vi "Teleop.vi"(10 "Match Info":T4={"Autonomous Elapsed Seconds"=0.0, "TeleOp Elapsed Seconds"=0.0, "Disabled Elapsed Seconds"=0.0, "Visited Autonomous"=FALSE, "Visited TeleOp"=FALSE, "Visited Disabled"=FALSE, "Autonomous Settings"={"Autonomous Style"=enum."Independent", "VI Refnum"=refnum}}, 11 "Call Context":T5) -> ()   [LabVIEW 2018]
doc: "This VI is called for each TeleOp packet received from the DS where the robot is not disabled. It is often used to read from the joysticks and update I/O or to update setpoints for timed control loops. It should complete and return within 20 milliseconds or it may miss DS packets."
uses:
  <vilib>/Rock Robotics/WPI/DriverStation/WPI_DriverStationDerivedRobotMode.ctl
  <vilib>/Rock Robotics/WPI/DriverStation/WPI_DriverStationMatch Info.ctl
  <vilib>/Rock Robotics/WPI/Solenoid/WPI_SolenoidValue.ctl
  <vilib>/Rock Robotics/WPI/ThirdParty/Phoenix-LabVIEW/Motor Controller/Controls/CTRE_Phoenix_MotorControl_ControlMode.ctl
  <vilib>/Rock Robotics/WPI/Utilities/WPI_GetSetVariantRefNum.vi
  <vilib>/Rock Robotics/WPI/Joystick/WPI_JoystickArcadeMapping.vi
  <vilib>/Rock Robotics/Network Tables/NT Write Boolean Array.vi
  <vilib>/Rock Robotics/Network Tables/NT Write Numeric Array.vi
  <vilib>/Rock Robotics/WPI/Solenoid/WPI_SolenoidSetEnum.vi
  <vilib>/Rock Robotics/WPI/ThirdParty/Phoenix-LabVIEW/Motor Controller/Get/CTRE_Phoenix_MotorController_GetSelectedSensorData.vi
  <vilib>/Rock Robotics/Network Tables/NT Read Boolean.vi
  <vilib>/Rock Robotics/Network Tables/NT Read Number.vi
  Toolbox/Simple Limit Switch/Limits(Switch+Encoder).vi
  Toolbox/Simple Limit Switch/Limits(DoubleEncoder).vi
panel:
  out "Wrist Out":dbl
  out "Wrist PID Out":dbl
  out "Elevator Out":dbl
  out "Elevator PID Out":dbl
  in  "Into Home Limit Is Pos (Encoder) Outer":bool
  in  "Into Home Limit Is Pos (Motor) Outer":bool=TRUE
  in  "Outer Limit":dbl format="%#_13g"
  in  "Into Home Limit is Pos Encoder (Horse)":bool=TRUE
  in  "Into Home Limit is Pos (Encoder) Wrist":bool
  in  "Into Home Limit Is Pos (Encoder) Elevator":bool
  in  "Elevator Home Encoder Limit":dbl format="%#_13g"
  in  "Elevator Encoder Limit":dbl=430000.0 format="%#_13g"
  in  "Reset Horse Encoder":bool
  out "OuterStageSwitch":bool
  out "Wrist After Dangerzone":T1(ring)
  out "Elevator  After Dangerzone":T2(ring)
  in  "Elevator Auto":bool=TRUE
  in  "Elevator Output Range":cluster{"output high":dbl, "output low":dbl}={"output high"=0.2, "output low"=-0.75}
  in  "Elevator PID Gains":T3={"proportional gain (Kc)"=-1e-05, "integral time (Ti, min)"=0.0, "derivative time (Td, min)"=0.0}
  in  "Elevator Setpoints":dbl[](array[numeric])=[1000.0, 100000.0, 250000.0, 250000.0, 270000.0, 480000.0]
  in  "Wrist Auto":bool=TRUE
  in  "Wrist Output Range":cluster{"output high":dbl, "output low":dbl}={"output high"=0.75, "output low"=-0.75}
  in  "Wrist PID Gains":T3={"proportional gain (Kc)"=-2e-05, "integral time (Ti, min)"=0.0, "derivative time (Td, min)"=0.0}
  in  "Wrist Setpoints":dbl[](array[numeric])=[150000.0, 150000.0, 45000.0, 45000.0, 0.0, 40000.0, 99000.0, 110000.0, 160000.0]
  in  "Into Home Limit Is Pos (Motor) Wrist":bool=TRUE
  out "Wrist Limit Switch":bool
  out "Elevator Limit Switch Top":bool
  in  "Into Home Limit Is Pos (Motor) Elevator":bool=TRUE
  in  "Intake Encoder Limit":dbl=170000.0 format="%#_13g"
  in  "Intake Home Encoder Limit":dbl format="%#_13g"
  in  "HorseDanger":i32=30000
  in  "Horse  Encoder Limit":dbl=-90000.0 format="%#_13g"
  in  "Into Home Limit Is Pos Motor (Horse)":bool
  out "Elevator Limit Switch":bool
  out "Elevator Encoder":i32=-47
  in  "Reset Elevator Encoder":bool
  out "Horse Encoder":i32
  in  "Reset Wrist Encoder":bool
  out "Intake Wrist Encoder":i32=4
  # "BETA POWER/DIRECTIONS\nElevator: Negative is up\nHorse: Negative is into robot\nOuter: Positive is down\nWrist: Negative is into robot"
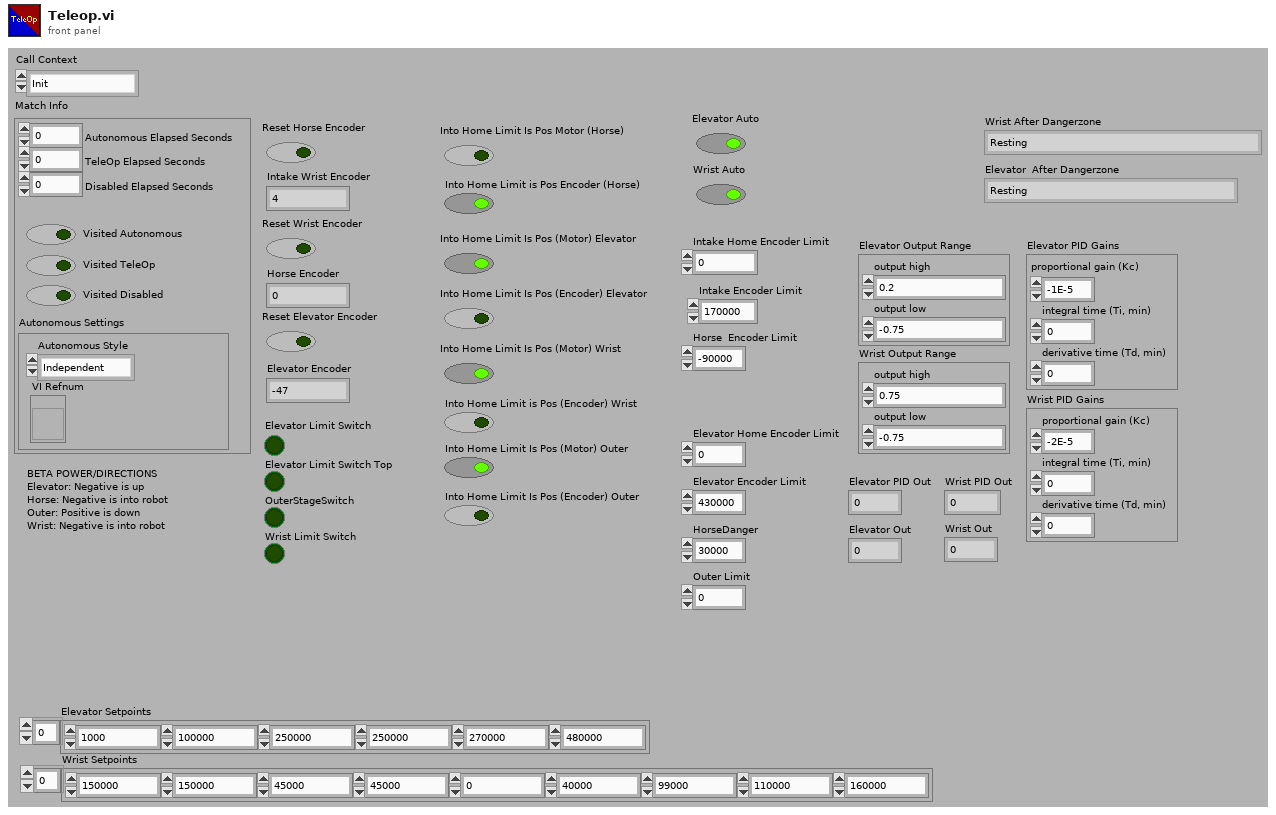
[diagram p1: front panel]
types:
  T1 = enum16{"Resting", "Hatch Ground Intake", "Hatch Place Low/Mid/CargoShip", "Hatch Place High", "Cargo Ground Intake", "Cargo Place Low/Mid", "Cargo Place High", "CargoShip Place Front", "CargoShip Place Back"}
  T2 = enum16{"Resting", "CargoShip Front", "CargoShip Back", "Cargo Mid", "Hatch Mid", "All High"}
  T3 = cluster{"proportional gain (Kc)":dbl, "integral time (Ti, min)":dbl, "derivative time (Td, min)":dbl}
  T4 = typedef "WPI_DriverStationMatch Info.ctl" = cluster{"Autonomous Elapsed Seconds":dbl, "TeleOp Elapsed Seconds":dbl, "Disabled Elapsed Seconds":dbl, "Visited Autonomous":bool, "Visited TeleOp":bool, "Visited Disabled":bool, "Autonomous Settings":cluster{"Autonomous Style":enum16{"Iterative", "Independent"}, "VI Refnum":refnum<vi>}}
  T5 = typedef "WPI_DriverStationDerivedRobotMode.ctl" = enum16{"Init", "Execute", "Stop"}
  T6 = typedef "CTRE_Phoenix_MotorControl_ControlMode.ctl" = u16
  T7 = typedef "WPI_SolenoidValue.ctl" = enum16{"Off", "On", "Forward", "Reverse"}
  T8 = cluster{"Intake Wheels Forwards":bool, "Elevator Shift":bool, "Intake Wheels Backwards":bool, "Drivetrain Shift":bool, "Elevator Outer Forwards":bool, "Elevator Outer Backwards":bool, "Horse Drive Climber":bool, "Horse Drive Pistons":bool, "Horse Drive Up":bool, "Horse Drive Down":bool, "Level 3 Climb":bool}
  T9 = enum16{"Intake Cargo", "Outtake Cargo", "Resting Cargo", "Reverse Cargo", "Intake Hatches", "Outtake Hatches", "Resting Hatches"}
  T10 = enum16{"Elevator Level 1", "Elevator Level 2", "Elevator Level 3"}
  T11 = typedef "WPI_JoystickDevRef.ctl" = cluster{"Device":T12}
  T12 = typedef "WPI_JoystickDeviceEnum.ctl" = enum16{"USB 0", "USB 1", "USB 2", "USB 3", "USB 4", "USB 5"}
  T13 = typedef "WPI_MotorControlDeviceRef.ctl" = cluster{"DeviceStatus":errorcluster, "Type":T14, "PWM":cluster{"PWM Channel":T15, "DeadBand":T16}, "CAN":cluster{"Device Number":u8, "SetOutput VI Ref":variant, "GetOutput VI Ref":variant, "Enable VI Ref":variant, "Disable VI Ref":variant, "Data":variant}, "Invert":bool, "DIO PWM":cluster{"PWM \"Enable\" Channel":T15, "DIOChannel":T17, "PWM Rate":dbl}}
  T14 = typedef "WPI_MotorControlType.ctl" = enum16{"PWM", "CAN", "DIO PWM"}
  T15 = typedef "FPGA_DIOPWMChannel.ctl" = enum8{"PWM 0", "PWM 1", "PWM 2", "PWM 3", "PWM 4", "PWM 5", "PWM 6", "PWM 7", "PWM 8", "PWM 9", "PWM MXP 0", "PWM MXP 1", "PWM MXP 2", "PWM MXP 3", "PWM MXP 4", "PWM MXP 5", "PWM MXP 6", "PWM MXP 7", "PWM MXP 8", "PWM MXP 9", "Invalid"}
  T16 = typedef "WPI_PWMDeadband.ctl" = cluster{"Name":string, "maxPositivePwm":i32, "minPositivePwm":i32, "centerPwm":i32, "maxNegativePwm":i32, "minNegativePwm":i32, "angularRange":u16}
  T17 = typedef "FPGA_DIOChannel.ctl" = enum8{"DIO 0", "DIO 1", "DIO 2", "DIO 3", "DIO 4", "DIO 5", "DIO 6", "DIO 7", "DIO 8", "DIO 9", "DIO MXP 0", "DIO MXP 1", "DIO MXP 2", "DIO MXP 3", "DIO MXP 4", "DIO MXP 5", "DIO MXP 6", "DIO MXP 7", "DIO MXP 8", "DIO MXP 9", "DIO MXP 10", "DIO MXP 11", "DIO MXP 12", "DIO MXP 13", "DIO MXP 14", "DIO MXP 15", "SPI Port CS1", "SPI Port CS2", "SPI Port CS3", "SPI Port MISO", "SPI Port MOSI", "Invalid"}
  T18 = cluster{"Elevator Setpoints":dbl[], "Wrist Setpoints":dbl[], "Horse Drive Setpoints":dbl[], "Wrist Gains":cluster{"proportional gain (Kc)":dbl, "integral time (Ti, min)":dbl, "derivative time (Td, min)":dbl}, "Wrist Power Limits":cluster{"output high":dbl, "output low":dbl}, "Horse Gains":cluster{"proportional gain (Kc)":dbl, "integral time (Ti, min)":dbl, "derivative time (Td, min)":dbl}, "Horse Power Limits":cluster{"output high":dbl, "output low":dbl}, "Elevator Gains":cluster{"proportional gain (Kc)":dbl, "integral time (Ti, min)":dbl, "derivative time (Td, min)":dbl}, "Elevator Power Limits":cluster{"output high":dbl, "output low":dbl}}
  T19 = enum16{"Resting", "CargoShip Front", "CargoShip Back", "Cargo Mid", "Hatch Mid", "All High", "Cargo Intake"}
  T20 = typedef "WPI_SolenoidDevRef.ctl" = cluster{"DevStatus":errorcluster, "Pneumatics Control Module":u8, "Forward Solenoid Channel":T21, "Reverse Solenoid Channel":T21}
  T21 = typedef "WPI_SolenoidChannel.ctl" = enum8{"Solenoid 0", "Solenoid 1", "Solenoid 2", "Solenoid 3", "Solenoid 4", "Solenoid 5", "Solenoid 6", "Solenoid 7", "Invalid"}
  T22 = typedef "WPI_SwitchDevRef.ctl" = cluster{"DevStatus":errorcluster, "DIO Channel":T17, "CntIndex":T23, "Normally Closed":bool}
  T23 = typedef "FPGA_CounterCtrSystemIndex.ctl" = enum8{"Ctr 0", "Ctr 1", "Ctr 2", "Ctr 3", "Ctr 4", "Ctr 5", "Ctr 6", "Ctr 7", "Invalid"}
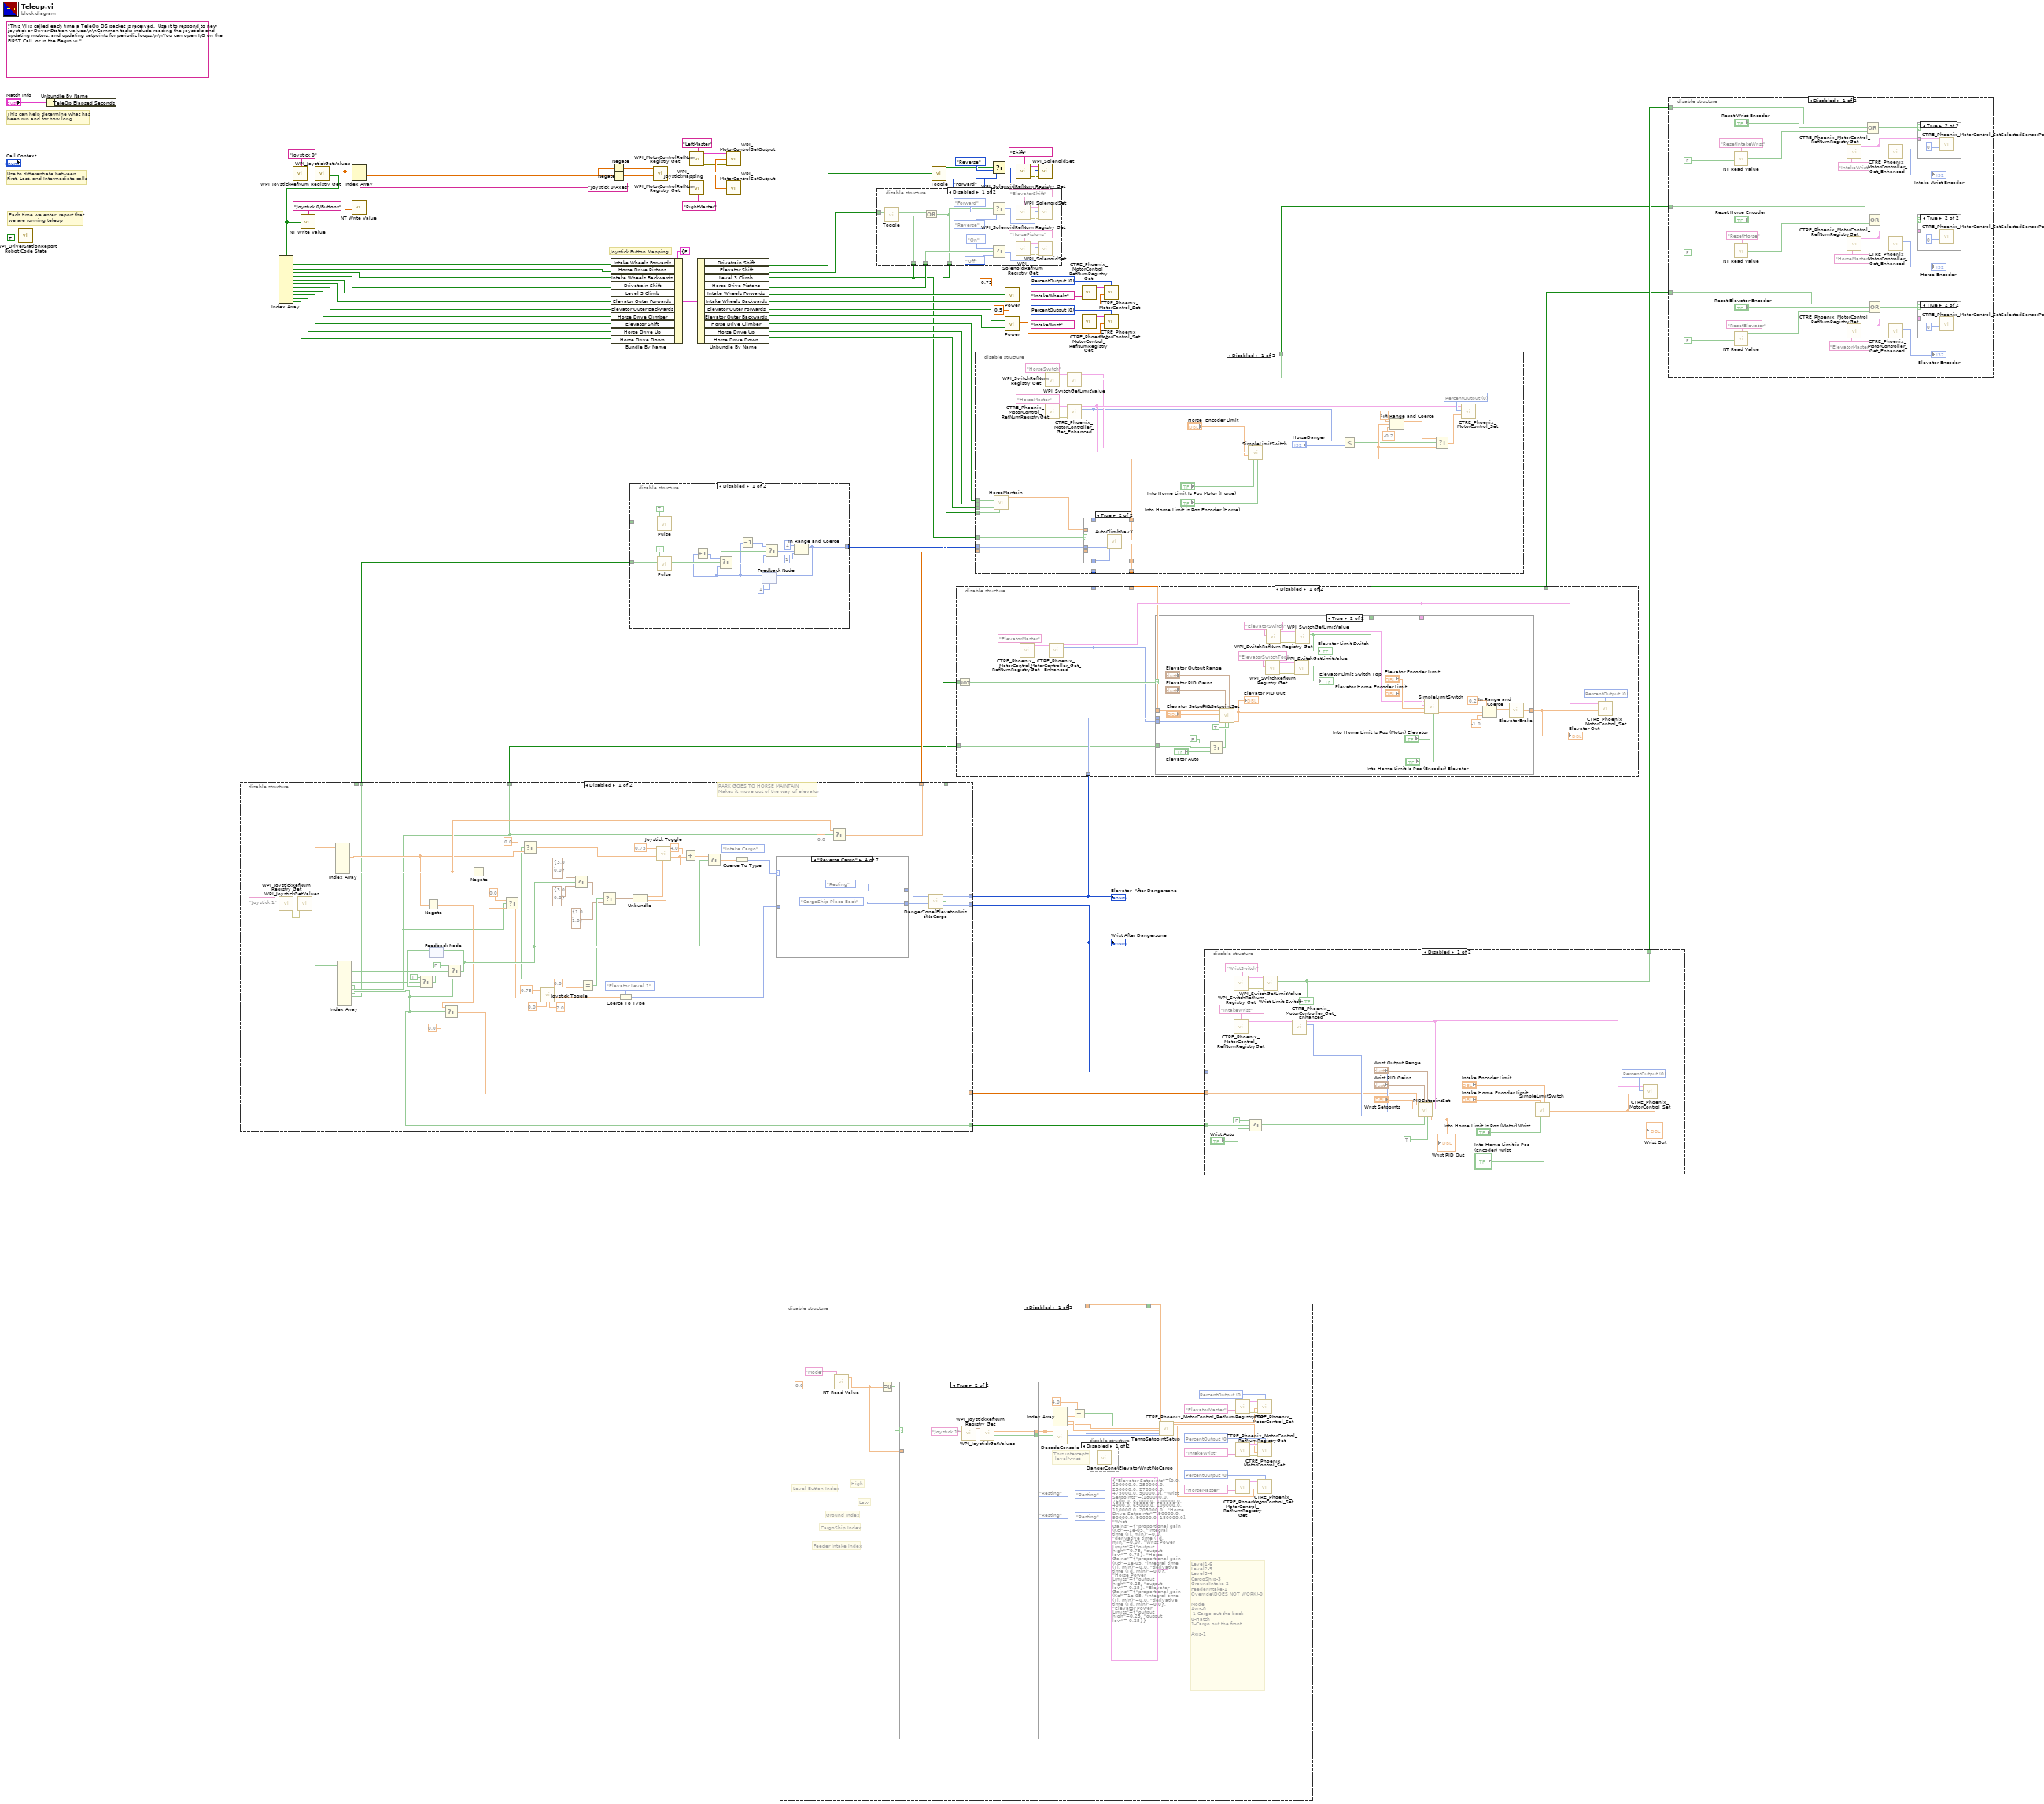
[diagram p0: block diagram]
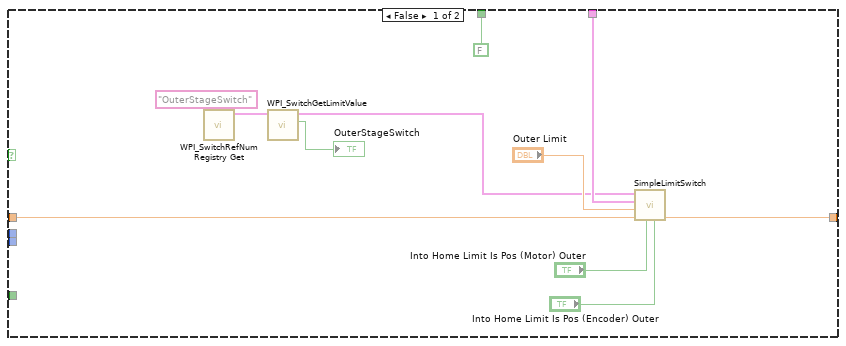
[diagram p3: hidden frame]
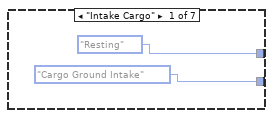
[diagram p5: hidden frame]
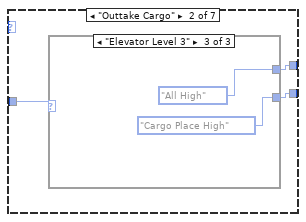
[diagram p6: hidden frame]
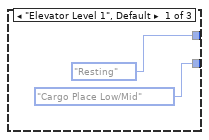
[diagram p7: hidden frame]
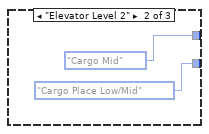
[diagram p8: hidden frame]
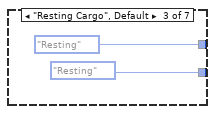
[diagram p9: hidden frame]
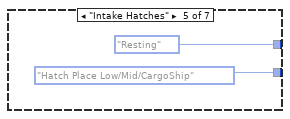
[diagram p10: hidden frame]
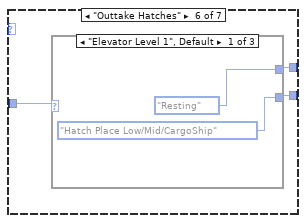
[diagram p11: hidden frame]
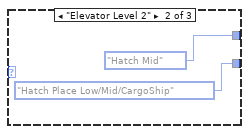
[diagram p12: hidden frame]
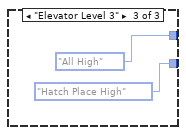
[diagram p13: hidden frame]
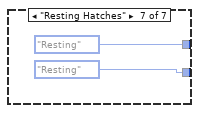
[diagram p14: hidden frame]
diagram:
  w4 = T6 0 items=["PercentOutput"=0, "Position"=1, "Velocity"=2, "Current"=3, "Follower"=5, "MotionProfile"=6, "MotionMagic"=7, "MotionProfileArc"=10, "Disabled"=15] ("Control Mode")
  w33 = T6 0 items=["PercentOutput"=0, "Position"=1, "Velocity"=2, "Current"=3, "Follower"=5, "MotionProfile"=6, "MotionMagic"=7, "MotionProfileArc"=10, "Disabled"=15] ("Control Mode")
  (unwired) "This VI is called each time a TeleOp DS packet is received.  Use it to respond to new joystick or Driver Station values.\n\nCommon tasks include reading the joysticks and updating motors, and updating setpoints for periodic loops.\n\nYou can open I/O on the FIRST Call, or in the Begin.vi."
  # "Joystick Button Mapping"
  # "Each time we enter, report that\nwe are running teleop"
  # "Use to differentiate between\nFirst, Last, and Intermediate calls"
  # "This can help determine what has\nbeen run and for how long"
  n1 = call <vilib>:"WPI_DriverStationReport Robot Code State.vi"("TeleOp"=TRUE ("Autonomous")) -> ()  [unwired: 10 in, 1 out]
  n2 = Unbundle By Name("Match Info") -> ()  [unwired: 1 out]
  n3 = disable-structure shown="Disabled" {
    disable-tunnel: [w130 _] -> w26
    disable-tunnel: [w118 _] -> w18
    disable-tunnel: [w91 _] -> w13
    disable-tunnel: [w90 _] -> w12
    disable-tunnel: [w89 _] -> w11
    disable-tunnel: [w80 _] -> w10
    disable-tunnel: [w79 _] -> w9
    disable-tunnel: [w78 _] -> w8
    disable-tunnel: [w77 _] -> w7
    frame Disabled {
      w121 = FALSE
      # "PARK GOES TO HORSE MAINTAIN\nMakes it move out of the way of elevator"
      n4 = call <vilib>:"WPI_JoystickRefNum Registry Get.vi"("refnum name"="Joystick 1") -> ("error out"=w129:errorcluster, "JoystickDevRef"=w128:T11)  [unwired: 9 in]
      n5 = call <vilib>:"WPI_JoystickGetValues.vi"("error in (no error)"=w129, "JoystickDevRef"=w128) -> ("Buttons"=w126:bool[], "Axes"=w127:dbl[])  [unwired: 5 in, 3 out]
      n6 = Index Array(array=w127) -> (element #2=w87:dbl, element #6=w92:dbl)  [unwired: 6 in, 4 out]
      n7 = Index Array(array=w126) -> (element #1=w125:bool, element #4=w81:bool, element #5=w79:bool, element #6=w80:bool, element #7=w77:bool, element #8=w78:bool)  [unwired: 10 in, 4 out]
      n8 = Negate(x=w87) -> (-x=w94:dbl)
      n9 = feedback #1(w121) -> (w123:bool)
      n10 = Select(t=TRUE, s=w81, f=w123) -> (s? t:f=w124:bool)
      n11 = Select(t=w94, s=w79, f=0.0) -> (s? t:f=w90:dbl)
      n12 = Select(t=w121, s=w125, f=w124) -> (s? t:f=w119:bool)
      n13 = feedback-in #1(w119) -> ()
      n14 = Negate(x=w92) -> (-x=w84:dbl)
      n15 = Select(t=0.0, s=w80, f=w84) -> (s? t:f=w83:dbl)
      n16 = Select(t=0.0, s=w79, f=w87) -> (s? t:f=w86:dbl)
      n17 = call "Joystick Toggle.vi"("Max"=2.0, "Min"=0.0, "Value"=w83, "Range"=0.75) -> ("Output"=w112:dbl)  [unwired: 7 in]
      n18 = Select(t=cluster{"Range":dbl, "Range 2":dbl} {"Range"=3.0, "Range 2"=0.0}, s=w119, f=cluster{"Range":dbl, "Range 2":dbl} {"Range"=3.0, "Range 2"=0.0}) -> (s? t:f=w105:cluster{"Range":dbl, "Range 2":dbl})
      n19 = Equal?(x=0.0, y=w112) -> (x = y?=w104:bool)
      n20 = Select(t=w105, s=w104, f=cluster{"Range":dbl, "Range 2":dbl} {"Range"=1.0, "Range 2"=1.0}) -> (s? t:f=w106:cluster{"Range":dbl, "Range 2":dbl})
      n21 = Coerce To Type(0:w112, 1:T10."Elevator Level 1") -> (2:w96:T10)
      n22 = Unbundle(w106) -> ("Range"=w108:dbl, "Range 2"=w107:dbl)
      n23 = call "Joystick Toggle.vi"("Max"=w107, "Min"=w108, "Value"=w86, "Range"=0.75) -> ("Output"=w99:dbl)  [unwired: 7 in]
      n24 = Add(x=4.0 ("y"), y=w99) -> (x+y=w100:dbl)
      n25 = Select(t=w100, s=w119, f=w99) -> (s? t:f=w102:dbl)
      n26 = Coerce To Type(0:w102, 1:T9."Intake Cargo") -> (2:w98:T9)
      n27 = case shown="\"Reverse Cargo\"" w98 {
        tunnel: [T1."Cargo Ground Intake" ("Wrist") w134 T1."Resting" ("Wrist") T1."CargoShip Place Back" ("Wrist") T1."Hatch Place Low/Mid/CargoShip" ("Wrist") w149 T1."Resting" ("Wrist")] -> w120
        tunnel: [T2."Resting" ("Elevator Level") w135 T2."Resting" ("Elevator Level") T2."Resting" ("Elevator Level") T2."Resting" ("Elevator Level") w150 T2."Resting" ("Elevator Level")] -> w117
        tunnel: w96 -> [_ w136 _ _ _ w151 _]
        frame "Intake Cargo" {
        }
        frame "Outtake Cargo" {
          n28 = case shown="\"Elevator Level 3\"" w136 {
            tunnel: [T2."Resting" ("Elevator Level") T2."Cargo Mid" ("Elevator Level") T2."All High" ("Elevator Level")] -> w135
            tunnel: [T1."Cargo Place Low/Mid" ("Wrist") T1."Cargo Place Low/Mid" ("Wrist") T1."Cargo Place High" ("Wrist")] -> w134
            frame "Elevator Level 1", Default {
            }
            frame "Elevator Level 2" {
            }
            frame "Elevator Level 3" {
            }
          }
        }
        frame "Resting Cargo", Default {
        }
        frame "Reverse Cargo" {
        }
        frame "Intake Hatches" {
        }
        frame "Outtake Hatches" {
          n29 = case shown="\"Elevator Level 1\", Default" w151 {
            tunnel: [T2."Resting" ("Elevator Level") T2."Hatch Mid" ("Elevator Level") T2."All High" ("Elevator Level")] -> w150
            tunnel: [T1."Hatch Place Low/Mid/CargoShip" ("Wrist") T1."Hatch Place Low/Mid/CargoShip" ("Wrist") T1."Hatch Place High" ("Wrist")] -> w149
            frame "Elevator Level 1", Default {
            }
            frame "Elevator Level 2" {
            }
            frame "Elevator Level 3" {
            }
          }
        }
        frame "Resting Hatches" {
        }
      }
      n30 = Select(t=w92, s=w80, f=0.0) -> (s? t:f=w91:dbl)
      n31 = call "DangerZone(ElevatorWrist)NoCargo.vi"("Wrist"=w120, "Level"=w117) -> ("Wrist"=w130:T1, "Park Horse"=w89:bool, "Level"=w118:T2)  [unwired: 1 in]
    }
    frame Enabled {
    }
  }
  "Elevator  After Dangerzone" <- w18
  "Wrist After Dangerzone" <- w26
  n32 = call <vilib>:"WPI_JoystickRefNum Registry Get.vi"("refnum name"="Joystick 0") -> ("error out"=w44:errorcluster, "JoystickDevRef"=w74:T11)  [unwired: 1 in, 8 out]
  n33 = call <vilib>:"WPI_JoystickGetValues.vi"("error in (no error)"=w44, "JoystickDevRef"=w74) -> ("Buttons"=w42:bool[], "Axes"=w70:dbl[])  [unwired: 5 in, 3 out]
  n34 = Index Array(array=w42) -> (element #1=w58:bool, element #2=w68:bool, element #3=w67:bool, element #4=w66:bool, element #5=w65:bool, element #6=w64:bool, element #7=w63:bool, element #8=w62:bool, element #9=w61:bool, element #10=w60:bool, element #11=w59:bool)  [unwired: 11 in]
  n35 = call-poly <vilib>:"NT Write Value.vi"("Boolean Array"=w42, "Name"="Joystick 0/Buttons") -> ()  [unwired: 9 in, 1 out]
  n36 = Index Array(array=w70) -> (element #1=w38:dbl, element #2=w41:dbl)  [unwired: 2 in]
  n37 = call-poly <vilib>:"NT Write Value.vi"("Numeric Array"=w70, "Name"="Joystick 0/Axes") -> ()  [unwired: 9 in, 1 out]
  n38 = Bundle By Name(cluster=T8 {"Intake Wheels Forwards"=FALSE, "Elevator Shift"=FALSE, "Intake Wheels Backwards"=FALSE, "Drivetrain Shift"=FALSE, "Elevator Outer Forwards"=FALSE, "Elevator Outer Backwards"=FALSE, "Horse Drive Climber"=FALSE, "Horse Drive Pistons"=FALSE, "Horse Drive Up"=FALSE, "Horse Drive Down"=FALSE, "Level 3 Climb"=FALSE} ("input cluster"), "Intake Wheels Forwards"=w58, "Horse Drive Pistons"=w68, "Intake Wheels Backwards"=w67, "Drivetrain Shift"=w66, "Level 3 Climb"=w65, "Elevator Outer Forwards"=w64, "Elevator Outer Backwards"=w63, "Horse Drive Climber"=w62, "Elevator Shift"=w61, "Horse Drive Up"=w60, "Horse Drive Down"=w59) -> (w57:T8)
  n39 = Negate(x=w38) -> (-x=w37:dbl)
  n40 = Negate(x=w41) -> (-x=w39:dbl)
  n41 = disable-structure shown="Disabled" {
    disable-tunnel: w8 -> [w165 _]
    disable-tunnel: w7 -> [w164 _]
    disable-tunnel: [w160 _] -> w6
    frame Disabled {
      n42 = call "Pulse.vi"("Input"=w164, "Rising Edge?"=TRUE) -> ("Output"=w168:bool)  [unwired: 9 in]
      n43 = call "Pulse.vi"("Input"=w165, "Rising Edge?"=TRUE) -> ("Output"=w173:bool)  [unwired: 9 in]
      n44 = feedback #2(1) -> (w166:i32)
      n45 = Increment(x=w166) -> (x+1=w172:i32)
      n46 = Select(t=w172, s=w173, f=w166) -> (s? t:f=w170:i32)
      n47 = Decrement(x=w166) -> (x-1=w167:i32)
      n48 = Select(t=w167, s=w168, f=w170) -> (s? t:f=w163:i32)
      n49 = In Range and Coerce(upper limit=4, x=w163, lower limit=1) -> (coerced(x)=w160:i32)  [unwired: 1 out]
      n50 = feedback-in #2(w160) -> ()
    }
    frame Enabled {
    }
  }
  n51 = call-poly <vilib>:"WPI_JoystickMapping.vi"("Y axis value"=w39, "X axis value"=w37) -> ("Right Motor Value"=w45:dbl, "Left Motor Value"=w46:dbl)  [unwired: 8 in]
  n52 = call <vilib>:"WPI_MotorControlRefNum Registry Get.vi"("refnum name"="LeftMaster") -> ("error out"=w24:errorcluster, "MotorControlDevRef"=w25:T13)  [unwired: 9 in]
  n53 = call <vilib>:"WPI_MotorControlRefNum Registry Get.vi"("refnum name"="RightMaster") -> ("error out"=w23:errorcluster, "MotorControlDevRef"=w22:T13)  [unwired: 9 in]
  n54 = Unbundle By Name(w57) -> ("Drivetrain Shift"=w40:bool, "Elevator Shift"=w16:bool, "Level 3 Climb"=w15:bool, "Horse Drive Pistons"=w31:bool, "Intake Wheels Forwards"=w50:bool, "Intake Wheels Backwards"=w49:bool, "Elevator Outer Forwards"=w48:bool, "Elevator Outer Backwards"=w47:bool, "Horse Drive Climber"=w27:bool, "Horse Drive Up"=w28:bool, "Horse Drive Down"=w29:bool)
  n55 = call <vilib>:"WPI_MotorControlSetOutput.vi"("error in (no error)"=w24, "Output"=w46, "MotorControlDevRef"=w25) -> ()  [unwired: 6 in, 3 out]
  n56 = call <vilib>:"WPI_MotorControlSetOutput.vi"("error in (no error)"=w23, "Output"=w45, "MotorControlDevRef"=w22) -> ()  [unwired: 6 in, 3 out]
  n57 = disable-structure shown="Disabled" {
    disable-tunnel: _ -> [w176 _]
    disable-tunnel: _ -> [w175 _]
    frame Disabled {
      w178 = T6 0 items=["PercentOutput"=0, "Position"=1, "Velocity"=2, "Current"=3, "Follower"=5, "MotionProfile"=6, "MotionMagic"=7, "MotionProfileArc"=10, "Disabled"=15] ("Control Mode")
      w185 = T6 0 items=["PercentOutput"=0, "Position"=1, "Velocity"=2, "Current"=3, "Follower"=5, "MotionProfile"=6, "MotionMagic"=7, "MotionProfileArc"=10, "Disabled"=15] ("Control Mode")
      w188 = T6 0 items=["PercentOutput"=0, "Position"=1, "Velocity"=2, "Current"=3, "Follower"=5, "MotionProfile"=6, "MotionMagic"=7, "MotionProfileArc"=10, "Disabled"=15] ("Control Mode")
      (unwired) T19."Resting" ("Elevator Level Select")
      (unwired) T19."Resting" ("Elevator Level Select")
      (unwired) T1."Resting" ("Wrist")
      (unwired) T1."Resting" ("Wrist")
      # "This intercepts\n level/wrist"
      # "Level1-6\nLevel2-5\nLevel3-4\nCargoShip-3\nGroundIntake-2\nFeederIntake-1\nOverride(DOES NOT WORK)-0\n\nMode\nAxis-0\n-1-Cargo out the back\n0-Hatch\n1-Cargo out the front\n\nAxis-1"
      # "CargoShip Index"
      # "Low"
      # "High"
      # "Feeder Intake Index"
      # "Ground Index"
      # "Level Button Index"
      n58 = call-poly <vilib>:"NT Read Value.vi"("Default Value"=0.0, "Name"="Mode") -> ("Numeric"=w200:dbl)  [unwired: 8 in, 1 out]
      n59 = Equal To 0?(x=w200) -> (x = 0?=w202:bool)
      n60 = case shown="True" w202 {
        tunnel: [w226 w239] -> w197
        tunnel: [w207 w238] -> w201
        tunnel: w200 -> [w206 _]
        frame False {
          n61 = case shown="4" w206 {
            tunnel: [0.0 0.0 1.0 -1.0 4.0] -> w205
            frame 0, Default {
            }
            frame 1 {
            }
            frame 2 {
            }
            frame 3 {
            }
            frame 4 {
            }
          }
          n62 = call-poly <vilib>:"NT Read Value.vi"("Default Value"=0.0, "Name"="ElevatorControl") -> ("Numeric"=w227:dbl)  [unwired: 8 in, 1 out]
          n63 = call-poly <vilib>:"NT Read Value.vi"("Default Value"=0.0, "Name"="WristControl") -> ("Numeric"=w228:dbl)  [unwired: 8 in, 1 out]
          n64 = call-poly <vilib>:"NT Read Value.vi"("Default Value"=FALSE, "Name"="Level3") -> ("Boolean"=w223:bool)  [unwired: 8 in, 1 out]
          n65 = call-poly <vilib>:"NT Read Value.vi"("Default Value"=FALSE, "Name"="Level2") -> ("Boolean"=w220:bool)  [unwired: 8 in, 1 out]
          n66 = call-poly <vilib>:"NT Read Value.vi"("Default Value"=FALSE, "Name"="Level1") -> ("Boolean"=w217:bool)  [unwired: 8 in, 1 out]
          n67 = call-poly <vilib>:"NT Read Value.vi"("Default Value"=FALSE, "Name"="IntakeGround") -> ("Boolean"=w214:bool)  [unwired: 8 in, 1 out]
          n68 = call-poly <vilib>:"NT Read Value.vi"("Default Value"=FALSE, "Name"="CargoShip") -> ("Boolean"=w211:bool)  [unwired: 8 in, 1 out]
          n69 = call-poly <vilib>:"NT Read Value.vi"("Default Value"=FALSE, "Name"="IntakeFeeder") -> ("Boolean"=w208:bool)  [unwired: 8 in, 1 out]
          n70 = Build Array(w205, w227, w228) -> (w226:dbl[])
          n71 = Build Array(w223, w220, w217, w214, w211, w208) -> (w207:bool[])
        }
        frame True {
          n72 = call <vilib>:"WPI_JoystickRefNum Registry Get.vi"("refnum name"="Joystick 1") -> ("JoystickDevRef"=w240:T11)  [unwired: 9 in, 1 out]
          n73 = call <vilib>:"WPI_JoystickGetValues.vi"("JoystickDevRef"=w240) -> ("Buttons"=w238:bool[], "Axes"=w239:dbl[])  [unwired: 6 in, 3 out]
        }
      }
      n74 = Index Array(array=w197) -> (element #1=w196:dbl, element #2=w193:dbl, element #3=w192:dbl)  [unwired: 3 in]
      n75 = call "DecodeConsole.vi"("Boolean Array"=w201, "Axis Array"=w197) -> ("Wrist"=w198:T1, "Elevator Level Select"=w199:T19)  [unwired: 8 in]
      n76 = Equal?(x=4.0, y=w196) -> (x = y?=w194:bool)
      n77 = disable-structure shown="Disabled" {
        frame Disabled {
          n78 = call "DangerZone(ElevatorWrist)NoCargo.vi"() -> ()  [unwired: 2 in, 2 out]
        }
        frame Enabled {
        }
      }
      n79 = call "TempSetpointSetup.vi"("Elevator Switch"=w175, "Enable Auto"=w194, "Elevator Manual Power"=w192, "Wrist Manual Power"=w193, "Horse Drive Manual Power"=w176, "Elevator Level Select"=w199, "Wrist"=w198, "Cluster"=T18 {"Elevator Setpoints"=[0.0, 100000.0, 250000.0, 250000.0, 270000.0, 475000.0, 50000.0], "Wrist Setpoints"=[180000.0, 7600.0, 82000.0, 100000.0, 4000.0, 69000.0, 100000.0, 110000.0, 205000.0], "Horse Drive Setpoints"=[90000.0, 90000.0, 90000.0, 180000.0], "Wrist Gains"={"proportional gain (Kc)"=-1e-05, "integral time (Ti, min)"=0.0, "derivative time (Td, min)"=0.0}, "Wrist Power Limits"={"output high"=0.75, "output low"=-0.75}, "Horse Gains"={"proportional gain (Kc)"=1e-05, "integral time (Ti, min)"=0.0, "derivative time (Td, min)"=0.0}, "Horse Power Limits"={"output high"=0.25, "output low"=-0.25}, "Elevator Gains"={"proportional gain (Kc)"=1e-05, "integral time (Ti, min)"=0.0, "derivative time (Td, min)"=0.0}, "Elevator Power Limits"={"output high"=0.25, "output low"=-0.25}}) -> ("Elevator Power Out"=w186:dbl, "Wrist Power Out"=w181:dbl, "Horse Drive Power Out"=w177:dbl)  [unwired: 17 in]
      n80 = call <vilib>:"CTRE_Phoenix_MotorControl_RefNumRegistryGet.vi"("refnum name"="ElevatorMaster") -> ("error out"=w187:errorcluster, "PhoenixMotorControlDevRef"=w189:T13)  [unwired: 9 in]
      n81 = call <vilib>:"CTRE_Phoenix_MotorControl_RefNumRegistryGet.vi"("refnum name"="IntakeWrist") -> ("error out"=w182:errorcluster, "PhoenixMotorControlDevRef"=w184:T13)  [unwired: 9 in]
      n82 = call <vilib>:"CTRE_Phoenix_MotorControl_RefNumRegistryGet.vi"("refnum name"="HorseMaster") -> ("PhoenixMotorControlDevRef"=w179:T13)  [unwired: 9 in, 1 out]
      n83 = call <vilib>:"CTRE_Phoenix_MotorControl_Set.vi"("error in (no error)"=w187, "Output"=w186, "Control Mode"=w188, "PhoenixMotorControlDevRef"=w189) -> ()  [unwired: 6 in, 2 out]
      n84 = call <vilib>:"CTRE_Phoenix_MotorControl_Set.vi"("error in (no error)"=w182, "Output"=w181, "Control Mode"=w185, "PhoenixMotorControlDevRef"=w184) -> ()  [unwired: 6 in, 2 out]
      n85 = call <vilib>:"CTRE_Phoenix_MotorControl_Set.vi"("Output"=w177, "Control Mode"=w178, "PhoenixMotorControlDevRef"=w179) -> ()  [unwired: 7 in, 2 out]
    }
    frame Enabled {
    }
  }
  n86 = disable-structure shown="Disabled" {
    disable-tunnel: w31 -> [w246 _]
    disable-tunnel: w16 -> [w245 _]
    disable-tunnel: w15 -> [w244 _]
    disable-tunnel: [w242 _] -> w14
    frame Disabled {
      n87 = call "Toggle.vi"("Input"=w245) -> ("Output"=w243:bool)  [unwired: 10 in]
      n88 = Or(x=w243, y=w244) -> (x .or. y?=w242:bool)
      n89 = Select(t=WPI_SolenoidValue."Forward" ("Value"), s=w242, f=WPI_SolenoidValue."Reverse" ("Value")) -> (s? t:f=w258:T7)
      n90 = Select(t=WPI_SolenoidValue."On" ("Value"), s=w246, f=WPI_SolenoidValue."Off" ("Value")) -> (s? t:f=w253:T7)
      n91 = call <vilib>:"WPI_SolenoidRefNum Registry Get.vi"("refnum name"="ElevatorShift") -> ("error out"=w247:errorcluster, "SolenoidDevRef"=w255:T20)  [unwired: 9 in]
      n92 = call <vilib>:"WPI_SolenoidRefNum Registry Get.vi"("refnum name"="HorsePistons") -> ("error out"=w248:errorcluster, "SolenoidDevRef"=w250:T20)  [unwired: 9 in]
      n93 = call-poly <vilib>:"WPI_SolenoidSet.vi"("error in (no error)"=w247, "Value"=w258, "SolenoidDevRef"=w255) -> ()  [unwired: 7 in, 2 out]
      n94 = call-poly <vilib>:"WPI_SolenoidSet.vi"("error in (no error)"=w248, "Value"=w253, "SolenoidDevRef"=w250) -> ()  [unwired: 7 in, 2 out]
    }
    frame Enabled {
    }
  }
  n95 = call "Toggle.vi"("Input"=w40) -> ("Output"=w52:bool)  [unwired: 10 in]
  n96 = disable-structure shown="Disabled" {
    disable-tunnel: w18 -> [w270 _]
    disable-tunnel: [w263 _] -> w17
    disable-tunnel: _ -> [w262 _]
    disable-tunnel: [w261 _] -> _
    disable-tunnel: w14 -> [w260 _]
    disable-tunnel: w10 -> [w259 _]
    frame Disabled {
      w268 = T6 0 items=["PercentOutput"=0, "Position"=1, "Velocity"=2, "Current"=3, "Follower"=5, "MotionProfile"=6, "MotionMagic"=7, "MotionProfileArc"=10, "Disabled"=15] ("Control Mode")
      n97 = Not(x=w260) -> (.not. x?=w265:bool)
      n98 = call <vilib>:"CTRE_Phoenix_MotorControl_RefNumRegistryGet.vi"("refnum name"="ElevatorMaster") -> ("PhoenixMotorControlDevRef"=w267:T13)  [unwired: 9 in, 1 out]
      n99 = call-poly <vilib>:"CTRE_Phoenix_MotorController_Get_Enhanced.vi"("PhoenixMotorControlDevRef"=w267) -> ("PhoenixMotorControlDevRef"=w266:T13, "Position (Raw Sensor Units)"=w261:i32)  [unwired: 11 in, 2 out]
      n100 = case shown="True" w265 {
        tunnel: w266 -> [w281 w308]
        tunnel: w261 -> [_ w302]
        tunnel: w270 -> [_ w301]
        tunnel: w262 -> [w271 w298]
        tunnel: [w277 w296] -> w264
        tunnel: [FALSE ("Switch Pressed") w286] -> w263
        tunnel: w259 -> [_ w282]
        frame False {
          n101 = call <vilib>:"WPI_SwitchRefNum Registry Get.vi"("refnum name"="OuterStageSwitch") -> ("SwitchDevRef"=w276:T22)  [unwired: 9 in, 1 out]
          n102 = call <vilib>:"WPI_SwitchGetLimitValue.vi"("SwitchDevRef"=w276) -> ("Switch Pressed"=→"OuterStageSwitch":bool, "SwitchDevRef"=w273:T22)  [unwired: 8 in, 1 out]
          n103 = call-poly "SimpleLimitSwitch.vi"("Into Home Limit Is Pos (Encoder)"="Into Home Limit Is Pos (Encoder) Outer", "Into Home Limit Is Pos (Motor)"="Into Home Limit Is Pos (Motor) Outer", "Power In"=w271, "Encoder Limit"="Outer Limit", "Motor Ref"=w281, "Limit Switch Ref"=w273) -> ("Power Out"=w277:dbl)  [unwired: 5 in]
        }
        frame True {
          n104 = Select(t=FALSE ("Update"), s=w282, f="Elevator Auto") -> (s? t:f=w283:bool)
          n105 = call "PIDSetpointSet.vi"("Update"=TRUE, "Output Range"="Elevator Output Range", "Auto"=w283, "PID Gains"="Elevator PID Gains", "Encoder Position"=w302, "Level"=w301, "Setpoints"="Elevator Setpoints", "Manual Power"=w298) -> ("Power Out"=w300:dbl)  [unwired: 3 in]
          "Elevator PID Out" <- w300
          n106 = call <vilib>:"WPI_SwitchRefNum Registry Get.vi"("refnum name"="ElevatorSwitchTop") -> ("error out"=w288:errorcluster, "SwitchDevRef"=w290:T22)  [unwired: 9 in]
          n107 = call <vilib>:"WPI_SwitchRefNum Registry Get.vi"("refnum name"="ElevatorSwitch") -> ("error out"=w293:errorcluster, "SwitchDevRef"=w294:T22)  [unwired: 9 in]
          n108 = call <vilib>:"WPI_SwitchGetLimitValue.vi"("error in (no error)"=w288, "SwitchDevRef"=w290) -> ("Switch Pressed"=→"Elevator Limit Switch Top":bool)  [unwired: 7 in, 2 out]
          n109 = call <vilib>:"WPI_SwitchGetLimitValue.vi"("error in (no error)"=w293, "SwitchDevRef"=w294) -> ("Switch Pressed"=w286:bool, "SwitchDevRef"=w291:T22)  [unwired: 7 in, 1 out]
          "Elevator Limit Switch" <- w286
          n110 = call-poly "SimpleLimitSwitch.vi"("Into Home Limit Is Pos (Encoder)"="Into Home Limit Is Pos (Encoder) Elevator", "Into Home Limit Is Pos (Motor)"="Into Home Limit Is Pos (Motor) Elevator", "Power In"=w300, "Encoder Limit"="Elevator Encoder Limit", "Motor Ref"=w308, "Limit Switch Ref"=w291) -> ("Power Out"=w311:dbl)  [unwired: 5 in]
          n111 = In Range and Coerce(upper limit=0.2, x=w311, lower limit=-1.0) -> (coerced(x)=w297:dbl)  [unwired: 1 out]
          n112 = call "ElevatorBrake.vi"("Power In"=w297) -> ("Power Out"=w296:dbl)
        }
      }
      "Elevator Out" <- w264
      n113 = call <vilib>:"CTRE_Phoenix_MotorControl_Set.vi"("Output"=w264, "Control Mode"=w268, "PhoenixMotorControlDevRef"=w266) -> ()  [unwired: 7 in, 2 out]
    }
    frame Enabled {
    }
  }
  n114 = disable-structure shown="Disabled" {
    disable-tunnel: w29 -> [w343 _]
    disable-tunnel: w28 -> [w342 _]
    disable-tunnel: w27 -> [w341 _]
    disable-tunnel: [w340 _] -> w19
    disable-tunnel: [w318 _] -> _
    disable-tunnel: _ -> [w317 _]
    disable-tunnel: w15 -> [w316 _]
    disable-tunnel: w13 -> [w315 _]
    disable-tunnel: w11 -> [w313 _]
    disable-tunnel: w6 -> [w312 _]
    frame Disabled {
      w336 = T6 0 items=["PercentOutput"=0, "Position"=1, "Velocity"=2, "Current"=3, "Follower"=5, "MotionProfile"=6, "MotionMagic"=7, "MotionProfileArc"=10, "Disabled"=15] ("Control Mode")
      n115 = call "HorseMantain.vi"("Park"=w313, "Negative"=w343, "Positive"=w342, "HorseToggle"=w341) -> ("Power"=w320:dbl)  [unwired: 7 in]
      n116 = call <vilib>:"WPI_SwitchRefNum Registry Get.vi"("refnum name"="HorseSwitch") -> ("error out"=w339:errorcluster, "SwitchDevRef"=w325:T22)  [unwired: 9 in]
      n117 = call <vilib>:"CTRE_Phoenix_MotorControl_RefNumRegistryGet.vi"("refnum name"="HorseMaster") -> ("error out"=w314:errorcluster, "PhoenixMotorControlDevRef"=w327:T13)  [unwired: 9 in]
      n118 = call <vilib>:"WPI_SwitchGetLimitValue.vi"("error in (no error)"=w339, "SwitchDevRef"=w325) -> ("Switch Pressed"=w340:bool, "SwitchDevRef"=w322:T22)  [unwired: 7 in, 1 out]
      n119 = call-poly <vilib>:"CTRE_Phoenix_MotorController_Get_Enhanced.vi"("PhoenixMotorControlDevRef"=w327, "error in"=w314) -> ("PhoenixMotorControlDevRef"=w326:T13, "Position (Raw Sensor Units)"=w321:i32)  [unwired: 10 in, 2 out]
      n120 = case shown="True" w316 {
        tunnel: w321 -> [_ w350]
        tunnel: [w344 w349] -> w319
        tunnel: [w345 w348] -> w318
        tunnel: w315 -> [w345 _]
        tunnel: w320 -> [w344 _]
        tunnel: w317 -> [_ w347]
        tunnel: w312 -> [_ w346]
        frame False {
        }
        frame True {
          n121 = call "AutoClimbNavX.vi"("Stage"=w346, "Elevator Encoder"=w347, "Horse Encoder"=w350) -> ("Elevator Output"=w348:dbl, "Horse Output"=w349:dbl)  [unwired: 7 in]
        }
      }
      n122 = call-poly "SimpleLimitSwitch.vi"("Into Home Limit Is Pos (Encoder)"="Into Home Limit is Pos Encoder (Horse)", "Into Home Limit Is Pos (Motor)"="Into Home Limit Is Pos Motor (Horse)", "Power In"=w319, "Encoder Limit"="Horse  Encoder Limit", "Motor Ref"=w326, "Limit Switch Ref"=w322) -> ("Power Out"=w330:dbl)  [unwired: 5 in]
      n123 = Less?(x=w321, y="HorseDanger") -> (x < y?=w328:bool)
      n124 = In Range and Coerce(upper limit=1.0, x=w330, lower limit=-0.2) -> (coerced(x)=w331:dbl)  [unwired: 1 out]
      n125 = Select(t=w331, s=w328, f=w330) -> (s? t:f=w329:dbl)
      n126 = call <vilib>:"CTRE_Phoenix_MotorControl_Set.vi"("Output"=w329, "Control Mode"=w336, "PhoenixMotorControlDevRef"=w326) -> ()  [unwired: 7 in, 2 out]
    }
    frame Enabled {
    }
  }
  n127 = Select(t=WPI_SolenoidValue."Reverse" ("Value"), s=w52, f=WPI_SolenoidValue."Forward" ("Value")) -> (s? t:f=w51:T7)
  n128 = call "Power.vi"("Positive Power"=0.75 ("Power"), "Negative"=w49, "Positive"=w50) -> ("Output"=w32:dbl)  [unwired: 8 in]
  n129 = call "Power.vi"("Positive Power"=0.5 ("Power"), "Negative"=w47, "Positive"=w48) -> ("Output"=w5:dbl)  [unwired: 8 in]
  n130 = call <vilib>:"WPI_SolenoidRefNum Registry Get.vi"("refnum name"="Shift") -> ("error out"=w43:errorcluster, "SolenoidDevRef"=w55:T20)  [unwired: 9 in]
  n131 = call-poly <vilib>:"WPI_SolenoidSet.vi"("error in (no error)"=w43, "Value"=w51, "SolenoidDevRef"=w55) -> ()  [unwired: 7 in, 2 out]
  n132 = call <vilib>:"CTRE_Phoenix_MotorControl_RefNumRegistryGet.vi"("refnum name"="IntakeWheels") -> ("PhoenixMotorControlDevRef"=w34:T13)  [unwired: 9 in, 1 out]
  n133 = call <vilib>:"CTRE_Phoenix_MotorControl_RefNumRegistryGet.vi"("refnum name"="IntakeWrist") -> ("PhoenixMotorControlDevRef"=w3:T13)  [unwired: 9 in, 1 out]
  n134 = call <vilib>:"CTRE_Phoenix_MotorControl_Set.vi"("Output"=w32, "Control Mode"=w33, "PhoenixMotorControlDevRef"=w34) -> ()  [unwired: 7 in, 2 out]
  n135 = call <vilib>:"CTRE_Phoenix_MotorControl_Set.vi"("Output"=w5, "Control Mode"=w4, "PhoenixMotorControlDevRef"=w3) -> ()  [unwired: 7 in, 2 out]
  n136 = disable-structure shown="Disabled" {
    disable-tunnel: [w366 _] -> w30
    disable-tunnel: w26 -> [w365 _]
    disable-tunnel: w12 -> [w355 _]
    disable-tunnel: w9 -> [w351 _]
    frame Disabled {
      w368 = T6 0 items=["PercentOutput"=0, "Position"=1, "Velocity"=2, "Current"=3, "Follower"=5, "MotionProfile"=6, "MotionMagic"=7, "MotionProfileArc"=10, "Disabled"=15] ("Control Mode")
      n137 = call <vilib>:"WPI_SwitchRefNum Registry Get.vi"("refnum name"="WristSwitch") -> ("error out"=w374:errorcluster, "SwitchDevRef"=w373:T22)  [unwired: 9 in]
      n138 = call <vilib>:"CTRE_Phoenix_MotorControl_RefNumRegistryGet.vi"("refnum name"="IntakeWrist") -> ("PhoenixMotorControlDevRef"=w369:T13)  [unwired: 9 in, 1 out]
      n139 = Select(t=FALSE ("Update"), s=w351, f="Wrist Auto") -> (s? t:f=w352:bool)
      n140 = call <vilib>:"WPI_SwitchGetLimitValue.vi"("error in (no error)"=w374, "SwitchDevRef"=w373) -> ("Switch Pressed"=w366:bool)  [unwired: 7 in, 2 out]
      "Wrist Limit Switch" <- w366
      n141 = call-poly <vilib>:"CTRE_Phoenix_MotorController_Get_Enhanced.vi"("PhoenixMotorControlDevRef"=w369) -> ("PhoenixMotorControlDevRef"=w367:T13, "Position (Raw Sensor Units)"=w370:i32)  [unwired: 11 in, 2 out]
      n142 = call "PIDSetpointSet.vi"("Update"=TRUE, "Output Range"="Wrist Output Range", "Auto"=w352, "PID Gains"="Wrist PID Gains", "Encoder Position"=w370, "Level"=w365, "Setpoints"="Wrist Setpoints", "Manual Power"=w355) -> ("Power Out"=w361:dbl)  [unwired: 3 in]
      "Wrist PID Out" <- w361
      n143 = call-poly "SimpleLimitSwitch.vi"("Into Home Limit is Pos (Encoder)"="Into Home Limit is Pos (Encoder) Wrist", "Encoder Limit"="Intake Encoder Limit", "Into Home Limit Is Pos (Motor)"="Into Home Limit Is Pos (Motor) Wrist", "Home Encoder Limit"="Intake Home Encoder Limit", "Power In"=w361, "Motor Ref"=w367) -> ("Power Out"=w372:dbl)  [unwired: 5 in]
      "Wrist Out" <- w372
      n144 = call <vilib>:"CTRE_Phoenix_MotorControl_Set.vi"("Output"=w372, "Control Mode"=w368, "PhoenixMotorControlDevRef"=w367) -> ()  [unwired: 7 in, 2 out]
    }
    frame Enabled {
    }
  }
  n145 = disable-structure shown="Disabled" {
    disable-tunnel: w30 -> [w381 _]
    disable-tunnel: w19 -> [w380 _]
    disable-tunnel: w17 -> [w376 _]
    frame Disabled {
      n146 = call-poly <vilib>:"NT Read Value.vi"("Default Value"=FALSE, "Name"="ResetIntakeWrist") -> ("Boolean"=w392:bool)  [unwired: 8 in, 1 out]
      n147 = call-poly <vilib>:"NT Read Value.vi"("Default Value"=FALSE, "Name"="ResetHorse") -> ("Boolean"=w389:bool)  [unwired: 8 in, 1 out]
      n148 = call-poly <vilib>:"NT Read Value.vi"("Default Value"=FALSE, "Name"="ResetElevator") -> ("Boolean"=w384:bool)  [unwired: 8 in, 1 out]
      n149 = call <vilib>:"CTRE_Phoenix_MotorControl_RefNumRegistryGet.vi"("refnum name"="IntakeWrist") -> ("PhoenixMotorControlDevRef"=w400:T13)  [unwired: 9 in, 1 out]
      n150 = call <vilib>:"CTRE_Phoenix_MotorControl_RefNumRegistryGet.vi"("refnum name"="HorseMaster") -> ("PhoenixMotorControlDevRef"=w399:T13)  [unwired: 9 in, 1 out]
      n151 = call <vilib>:"CTRE_Phoenix_MotorControl_RefNumRegistryGet.vi"("refnum name"="ElevatorMaster") -> ("PhoenixMotorControlDevRef"=w394:T13)  [unwired: 9 in, 1 out]
      n152 = Compound Arithmetic op=OR(w381, "Reset Wrist Encoder", w392) -> (w377:bool)
      n153 = Compound Arithmetic op=OR(w380, "Reset Horse Encoder", w389) -> (w378:bool)
      n154 = Compound Arithmetic op=OR(w376, "Reset Elevator Encoder", w384) -> (w379:bool)
      n155 = call-poly <vilib>:"CTRE_Phoenix_MotorController_Get_Enhanced.vi"("PhoenixMotorControlDevRef"=w400) -> ("Position (Raw Sensor Units)"=→"Intake Wrist Encoder":i32)  [unwired: 11 in, 3 out]
      n156 = call-poly <vilib>:"CTRE_Phoenix_MotorController_Get_Enhanced.vi"("PhoenixMotorControlDevRef"=w399) -> ("Position (Raw Sensor Units)"=→"Horse Encoder":i32)  [unwired: 11 in, 3 out]
      n157 = call-poly <vilib>:"CTRE_Phoenix_MotorController_Get_Enhanced.vi"("PhoenixMotorControlDevRef"=w394) -> ("Position (Raw Sensor Units)"=→"Elevator Encoder":i32)  [unwired: 11 in, 3 out]
      n158 = case shown="True" w377 {
        tunnel: w400 -> [_ w408]
        frame False {
        }
        frame True {
          n159 = call <vilib>:"CTRE_Phoenix_MotorControl_SetSelectedSensorPosition.vi"("New Sensor Position"=0, "PhoenixMotorControlDevRef"=w408) -> ()  [unwired: 8 in, 2 out]
        }
      }
      n160 = case shown="True" w378 {
        tunnel: w399 -> [_ w406]
        frame False {
        }
        frame True {
          n161 = call <vilib>:"CTRE_Phoenix_MotorControl_SetSelectedSensorPosition.vi"("New Sensor Position"=0, "PhoenixMotorControlDevRef"=w406) -> ()  [unwired: 8 in, 2 out]
        }
      }
      n162 = case shown="True" w379 {
        tunnel: w394 -> [_ w404]
        frame False {
        }
        frame True {
          n163 = call <vilib>:"CTRE_Phoenix_MotorControl_SetSelectedSensorPosition.vi"("New Sensor Position"=0, "PhoenixMotorControlDevRef"=w404) -> ()  [unwired: 8 in, 2 out]
        }
      }
    }
    frame Enabled {
    }
  }
